vi "Build Dqmh Module Relationship Sub Graph.vi"(7 "Link Type":T1, 9 "Module Name":string, 10 "Caller Names":string[](array[string]), 11 "Graph in":refnum<class "Graph.lvclass">) -> (1 "Specific Edge Shape":T2[](array[typedef]), 2 "Specific Node Shape":T3[](array[typedef]), 3 "Graph out":refnum<class "Graph.lvclass">)   [LabVIEW 2021, in "TAF Proj Document Type.lvlib" / "Dqmh Modules Overview.lvclass"]
uses:
  <vilib>/Wovalab/AntiDoc/Document Type/Add-ons/LabVIEW TAF Project/Dqmh Modules Overview/Dqmh Modules Overview.lvclass
  <vilib>/Wovalab/AntiDoc/GraphBuilder/Graph/Graph.lvclass
  <vilib>/Wovalab/AntiDoc/GraphBuilder/Renderer/Graphviz/Specific Node Shape Def.ctl
  <vilib>/Wovalab/AntiDoc/GraphBuilder/Shapes/Node/Graphviz/Graphviz Node Shape.lvclass
  <vilib>/Wovalab/AntiDoc/GraphBuilder/Renderer/Graphviz/Specific Edge Shape Def.ctl
  <vilib>/Wovalab/AntiDoc/GraphBuilder/Shapes/Edge/Graphviz/Graphviz Edge Shape.lvclass
  <vilib>/Wovalab/AntiDoc/Document Type/Add-ons/LabVIEW TAF Project/Dqmh Modules Overview/Link Type--enum.ctl
  <vilib>/Wovalab/AntiDoc/Document Type/Add-ons/LabVIEW TAF Project/Shared/Dqmh Event Module Link Type.ctl
  <vilib>/Wovalab/AntiDoc/Document Type/Add-ons/LabVIEW TAF Project/TAF Proj Document Type.lvlib
  <vilib>/Wovalab/AntiDoc/GraphBuilder/Renderer/Graphviz/Graphviz.lvclass
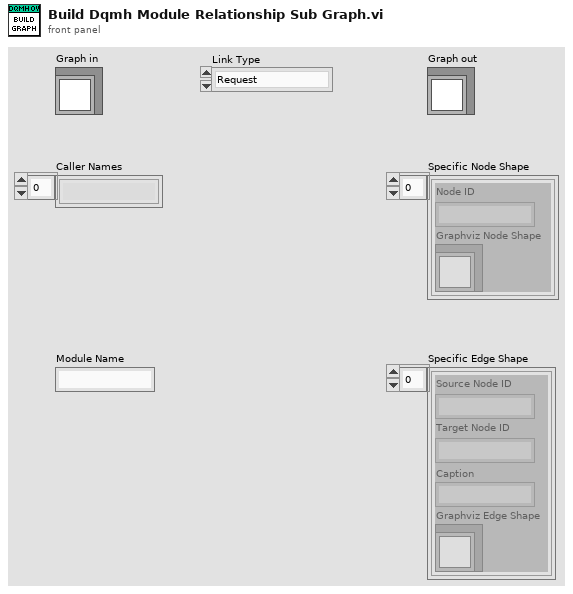
[diagram p1: front panel]
types:
  T1 = typedef "TAF Proj Document Type.lvlib/Dqmh Modules Overview.lvclass/Link Type--enum.ctl" = enum16{"Request", "Broadcast", "Request With Reply"}
  T2 = typedef "GraphBuilder.lvlib/Graphviz.lvclass/Specific Edge Shape Def.ctl" = cluster{"Source Node ID":string, "Target Node ID":string, "Caption":string, "Graphviz Edge Shape":refnum<class "Graphviz Edge Shape.lvclass">}
  T3 = typedef "GraphBuilder.lvlib/Graphviz.lvclass/Specific Node Shape Def.ctl" = cluster{"Node ID":string, "Graphviz Node Shape":refnum<class "Graphviz Node Shape.lvclass">}
  T4 = typedef "TAF Proj Document Type.lvlib/Dqmh Event Module Link Type.ctl" = enum16{"Request", "Request With Reply", "Broadcast", "Registred Broadcast", "Used Requests", "Used Requests With Reply"}
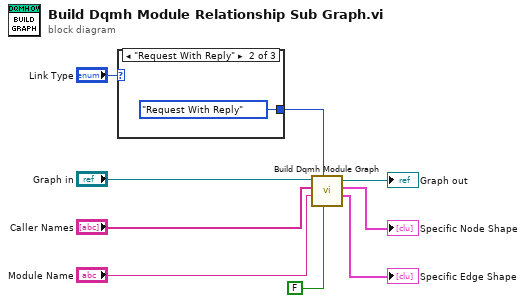
[diagram p0: block diagram]
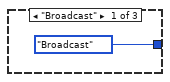
[diagram p2: hidden frame]
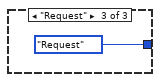
[diagram p3: hidden frame]
diagram:
  n1 = case shown="\"Request With Reply\"" "Link Type" {
    tunnel: [Dqmh_Event_Module_Link_Type."Broadcast" ("Link Type") Dqmh_Event_Module_Link_Type."Request With Reply" ("Link Type") Dqmh_Event_Module_Link_Type."Request" ("Link Type")] -> w5
    frame "Broadcast" {
    }
    frame "Request With Reply" {
    }
    frame "Request" {
    }
  }
  n2 = call <vilib>:"Build Dqmh Module Graph.vi"("Draw API Tester Link"=FALSE, "Link Type"=w5, "Module Name"="Module Name", "Link Name"="Caller Names", "Graph in"="Graph in") -> ("Specific Edge Shape"=→"Specific Edge Shape":T2[], "Specific Node Shape"=→"Specific Node Shape":T3[], "Graph out"=→"Graph out":refnum<class "Graph.lvclass">)  [unwired: 4 in]
